vi "Teleop.vi"(10 "Match Info":T1={"Autonomous Elapsed Seconds"=0.0, "TeleOp Elapsed Seconds"=0.0, "Disabled Elapsed Seconds"=0.0, "Visited Autonomous"=FALSE, "Visited TeleOp"=FALSE, "Visited Disabled"=FALSE, "Autonomous Settings"={"Autonomous Style"=enum."Independent", "VI Refnum"=refnum}}, 11 "Call Context":T2) -> ()   [LabVIEW 2015]
doc: "This VI is called for each TeleOp packet received from the DS where the robot is not disabled. It is often used to read from the joysticks and update I/O or to update setpoints for timed control loops. It should complete and return within 20 milliseconds or it may miss DS packets."
uses:
  <vilib>/Rock Robotics/WPI/DriverStation/WPI_DriverStationDerivedRobotMode.ctl
  <vilib>/Rock Robotics/WPI/DriverStation/WPI_DriverStationMatch Info.ctl
  <vilib>/Rock Robotics/WPI/Utilities/WPI_GetSetVariantRefNum.vi
  <vilib>/Rock Robotics/Network Tables/NT Write Boolean Array.vi
  <vilib>/Rock Robotics/Network Tables/NT Write Numeric Array.vi
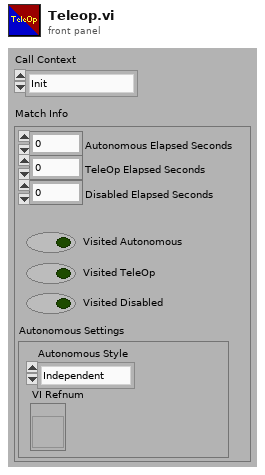
[diagram p1: front panel]
types:
  T1 = typedef "WPI_DriverStationMatch Info.ctl" = cluster{"Autonomous Elapsed Seconds":dbl, "TeleOp Elapsed Seconds":dbl, "Disabled Elapsed Seconds":dbl, "Visited Autonomous":bool, "Visited TeleOp":bool, "Visited Disabled":bool, "Autonomous Settings":cluster{"Autonomous Style":enum16{"Iterative", "Independent"}, "VI Refnum":refnum<vi>}}
  T2 = typedef "WPI_DriverStationDerivedRobotMode.ctl" = enum16{"Init", "Execute", "Stop"}
  T3 = typedef "WPI_JoystickDevRef.ctl" = cluster{"Device":T4}
  T4 = typedef "WPI_JoystickDeviceEnum.ctl" = enum16{"USB 0", "USB 1", "USB 2", "USB 3", "USB 4", "USB 5"}
  T5 = typedef "WPI_RobotDriveDevRef.ctl" = cluster{"DevStatus":errorcluster, "Motors[]":T6[], "Square Inputs":bool, "Max Output":dbl}
  T6 = typedef "WPI_MotorControlDeviceRef.ctl" = cluster{"DeviceStatus":errorcluster, "Type":T7, "PWM":cluster{"PWM Channel":T8, "DeadBand":T9}, "CAN":cluster{"Device Number":u8, "Control Mode":T10, "Semaphore":T11, "Max Vout":dbl, "TalonSRX Control Mode":T12}, "Invert":bool}
  T7 = typedef "WPI_MotorControlType.ctl" = enum16{"PWM", "CAN", "CANTalonSRX"}
  T8 = typedef "FPGA_DIOPWMChannel.ctl" = enum8{"PWM 0", "PWM 1", "PWM 2", "PWM 3", "PWM 4", "PWM 5", "PWM 6", "PWM 7", "PWM 8", "PWM 9", "PWM MXP 0", "PWM MXP 1", "PWM MXP 2", "PWM MXP 3", "PWM MXP 4", "PWM MXP 5", "PWM MXP 6", "PWM MXP 7", "PWM MXP 8", "PWM MXP 9", "Invalid"}
  T9 = typedef "WPI_PWMDeadband.ctl" = cluster{"Name":string, "maxPositivePwm":i32, "minPositivePwm":i32, "centerPwm":i32, "maxNegativePwm":i32, "minNegativePwm":i32, "angularRange":u16}
  T10 = typedef "WPI_CANJaguar_ControlMode.ctl" = enum8{"Percent VBus", "Current", "Speed", "Position", "Voltage"}
  T11 = typedef "Semaphore RefNum" = refnum<k1>
  T12 = typedef "WPI_CANTalonSRX_APIControlMode.ctl" = enum8{"Percent VBus", "Speed", "Position", "Slave", "Unchanged / Invalid", "Voltage Compensation", "Current", "Motion Profile"}
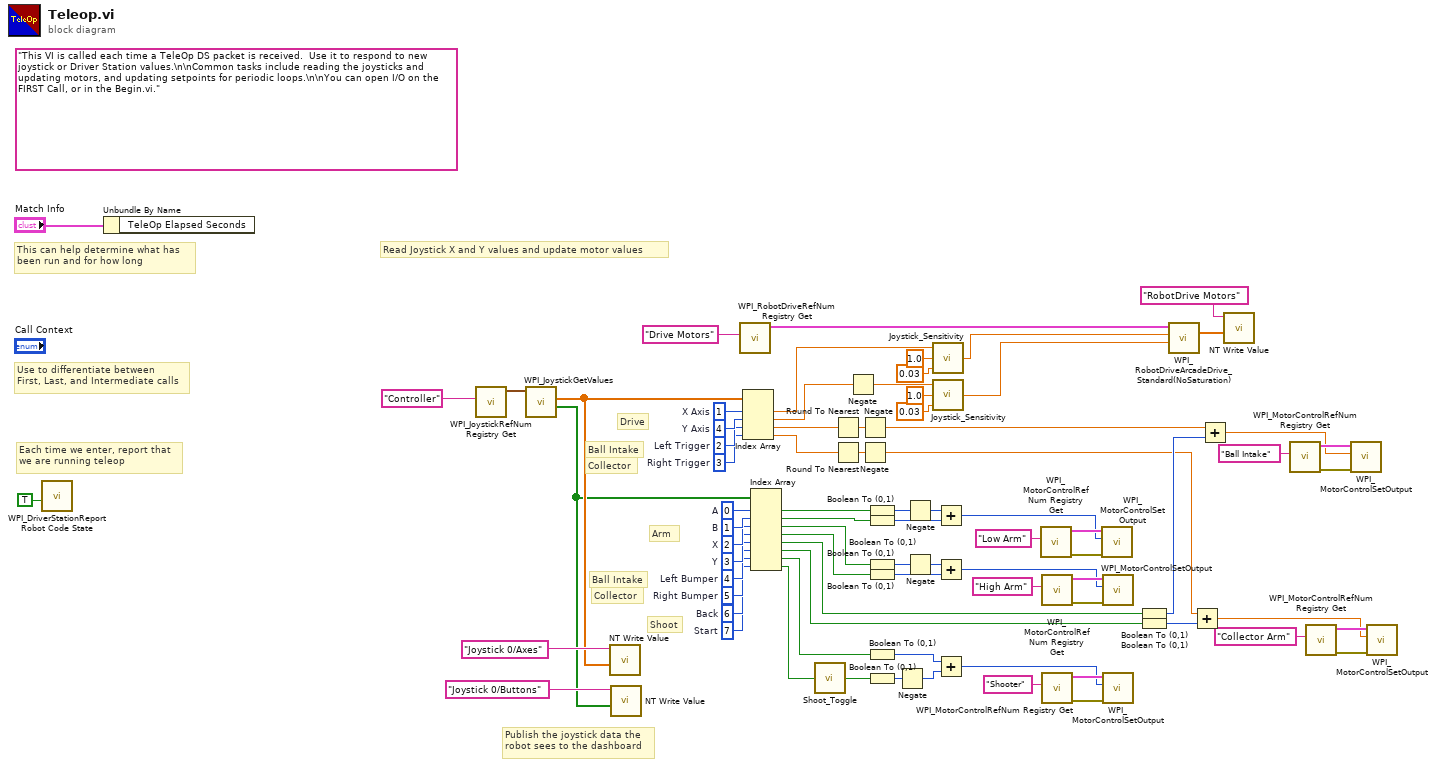
[diagram p0: block diagram]
diagram:
  w19 = 7  # Start
  w25 = 6  # Back
  w63 = 3  # Right Trigger
  w64 = 2  # Left Trigger
  w26 = 5  # Right Bumper
  w27 = 4  # Left Bumper
  w31 = 0  # A
  w30 = 1  # B
  w29 = 2  # X
  w28 = 3  # Y
  w65 = 4  # Y Axis
  w67 = 1  # X Axis
  (unwired) "This VI is called each time a TeleOp DS packet is received.  Use it to respond to new joystick or Driver Station values.\n\nCommon tasks include reading the joysticks and updating motors, and updating setpoints for periodic loops.\n\nYou can open I/O on the FIRST Call, or in the Begin.vi."
  # "Ball Intake"
  # "Collector"
  # "Shoot"
  # "Drive"
  # "Ball Intake"
  # "Collector"
  # "Arm"
  # "Publish the joystick data the\nrobot sees to the dashboard"
  # "Each time we enter, report that\nwe are running teleop"
  # "Use to differentiate between\nFirst, Last, and Intermediate calls"
  # "This can help determine what has\nbeen run and for how long"
  # "Read Joystick X and Y values and update motor values"
  n1 = call <vilib>:"WPI_DriverStationReport Robot Code State.vi"("TeleOp"=TRUE ("Autonomous")) -> ()  [unwired: 10 in, 1 out]
  n2 = Unbundle By Name("Match Info") -> ()  [unwired: 1 out]
  n3 = call <vilib>:"WPI_JoystickRefNum Registry Get.vi"("refnum name"="Controller") -> ("JoystickDevRef"=w75:T3)  [unwired: 1 in, 9 out]
  n4 = call <vilib>:"WPI_JoystickGetValues.vi"("JoystickDevRef"=w75) -> ("Buttons"=w66:bool[], "Axes"=w70:dbl[])  [unwired: 6 in, 3 out]
  n5 = call-poly <vilib>:"NT Write Value.vi"("Numeric Array"=w70, "Name"="Joystick 0/Axes") -> ()  [unwired: 9 in, 1 out]
  n6 = call-poly <vilib>:"NT Write Value.vi"("Boolean Array"=w66, "Name"="Joystick 0/Buttons") -> ()  [unwired: 9 in, 1 out]
  n7 = call <vilib>:"WPI_RobotDriveRefNum Registry Get.vi"("refnum name"="Drive Motors") -> ("RobotDriveDevRef"=w77:T5)  [unwired: 1 in, 9 out]
  n8 = Index Array(array=w70, index #1=w67, index #2=w65, index #3=w64, index #4=w63) -> (element #1=w10:dbl, element #2=w73:dbl, element #3=w62:dbl, element #4=w61:dbl)
  n9 = Index Array(array=w66, index #1=w31, index #2=w30, index #3=w29, index #4=w28, index #5=w27, index #6=w26, index #7=w25, index #8=w19) -> (element #1=w24:bool, element #2=w23:bool, element #3=w22:bool, element #4=w21:bool, element #5=w6:bool, element #6=w20:bool, element #7=w18:bool, element #8=w17:bool)
  n10 = call "Shoot_Toggle.vi"("Input"=w17) -> ("Output"=w57:bool)
  n11 = Round To Nearest(number=w62) -> (nearest integer value=w53:dbl)
  n12 = Round To Nearest(number=w61) -> (nearest integer value=w7:dbl)
  n13 = Negate(x=w73) -> (-x=w13:dbl)
  n14 = Negate(x=w53) -> (-x=w46:dbl)
  n15 = Negate(x=w7) -> (-x=w3:dbl)
  n16 = Boolean To (0,1)(Boolean=w24) -> (0, 1=w34:i16)
  n17 = Boolean To (0,1)(Boolean=w23) -> (0, 1=w35:i16)
  n18 = Boolean To (0,1)(Boolean=w22) -> (0, 1=w37:i16)
  n19 = Boolean To (0,1)(Boolean=w21) -> (0, 1=w39:i16)
  n20 = Boolean To (0,1)(Boolean=w18) -> (0, 1=w15:i16)
  n21 = Boolean To (0,1)(Boolean=w57) -> (0, 1=w56:i16)
  n22 = Negate(x=w56) -> (-x=w16:i16)
  n23 = Negate(x=w34) -> (-x=w36:i16)
  n24 = Negate(x=w37) -> (-x=w38:i16)
  n25 = call "Joystick_Sensitivity.vi"("Deadband"=0.03, "Ramp"=1.0, "Input"=w10) -> ("Output"=w9:dbl)
  n26 = call "Joystick_Sensitivity.vi"("Deadband"=0.03, "Ramp"=1.0, "Input"=w13) -> ("Output"=w12:dbl)
  n27 = Add(x=w36, y=w35) -> (x+y=w32:i16)
  n28 = Add(x=w38, y=w39) -> (x+y=w33:i16)
  n29 = Add(x=w15, y=w16) -> (x+y=w14:i16)
  n30 = call <vilib>:"WPI_MotorControlRefNum Registry Get.vi"("refnum name"="Low Arm") -> ("error out"=w41:errorcluster, "MotorControlDevRef"=w40:T6)  [unwired: 9 in]
  n31 = call <vilib>:"WPI_MotorControlRefNum Registry Get.vi"("refnum name"="High Arm") -> ("error out"=w44:errorcluster, "MotorControlDevRef"=w43:T6)  [unwired: 9 in]
  n32 = call <vilib>:"WPI_MotorControlRefNum Registry Get.vi"("refnum name"="Shooter") -> ("error out"=w59:errorcluster, "MotorControlDevRef"=w58:T6)  [unwired: 9 in]
  n33 = call <vilib>:"WPI_MotorControlSetOutput.vi"("error in (no error)"=w41, "Output"=w32, "MotorControlDevRef"=w40) -> ()  [unwired: 6 in, 3 out]
  n34 = call <vilib>:"WPI_MotorControlSetOutput.vi"("error in (no error)"=w44, "Output"=w33, "MotorControlDevRef"=w43) -> ()  [unwired: 6 in, 3 out]
  n35 = call <vilib>:"WPI_MotorControlSetOutput.vi"("error in (no error)"=w59, "Output"=w14, "MotorControlDevRef"=w58) -> ()  [unwired: 6 in, 3 out]
  n36 = Boolean To (0,1)(Boolean=w6) -> (0, 1=w5:i16)
  n37 = Boolean To (0,1)(Boolean=w20) -> (0, 1=w4:i16)
  n38 = call <vilib>:"WPI_RobotDriveArcadeDrive_Standard(NoSaturation).vi"("Y axis value"=w12, "X axis value"=w9, "RobotDriveDevRef"=w77) -> ("Motor Values"=w69:dbl[])  [unwired: 1 in, 7 out]
  n39 = Add(x=w3, y=w4) -> (x+y=w47:dbl)
  n40 = Add(x=w46, y=w5) -> (x+y=w51:dbl)
  n41 = call-poly <vilib>:"NT Write Value.vi"("Numeric Array"=w69, "Name"="RobotDrive Motors") -> ()  [unwired: 9 in, 1 out]
  n42 = call <vilib>:"WPI_MotorControlRefNum Registry Get.vi"("refnum name"="Ball Intake") -> ("error out"=w55:errorcluster, "MotorControlDevRef"=w54:T6)  [unwired: 9 in]
  n43 = call <vilib>:"WPI_MotorControlRefNum Registry Get.vi"("refnum name"="Collector Arm") -> ("error out"=w49:errorcluster, "MotorControlDevRef"=w48:T6)  [unwired: 9 in]
  n44 = call <vilib>:"WPI_MotorControlSetOutput.vi"("error in (no error)"=w55, "Output"=w51, "MotorControlDevRef"=w54) -> ()  [unwired: 6 in, 3 out]
  n45 = call <vilib>:"WPI_MotorControlSetOutput.vi"("error in (no error)"=w49, "Output"=w47, "MotorControlDevRef"=w48) -> ()  [unwired: 6 in, 3 out]
